vi "downloadSaved.vi"(8 "error in":errorcluster) -> (0 "error out":errorcluster, 3 "OK?":bool)   [LabVIEW 2024]
uses:
  session.vi
  user_name.vi
  <vilib>/httpClient/LabVIEWHTTPClient.lvlib
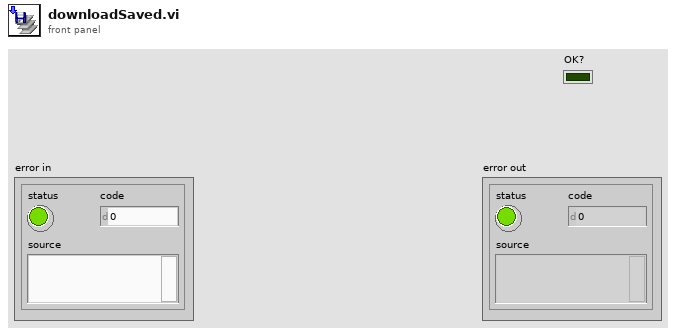
[diagram p1: front panel]
types:
  T1 = typedef "LabVIEWHTTPClient.lvlib/ClientHandle.ctl" = refnum<k1>
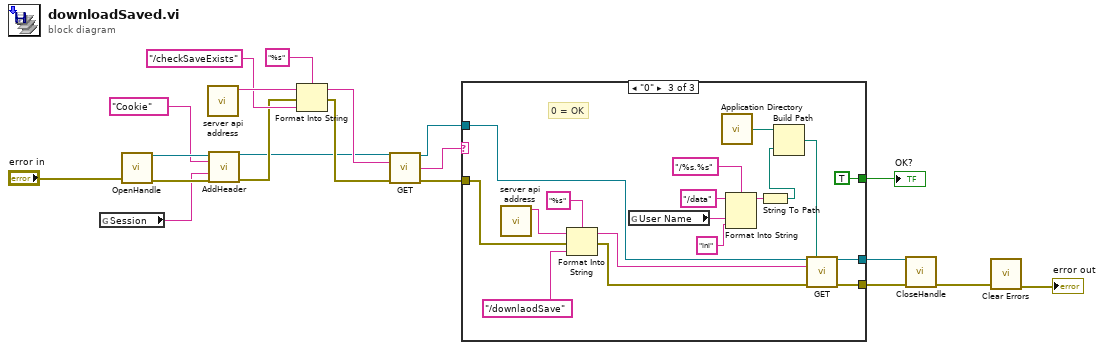
[diagram p0: block diagram]
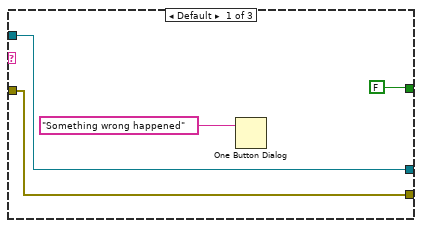
[diagram p2: hidden frame]
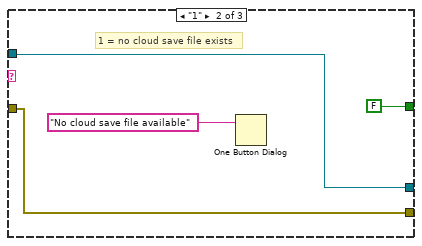
[diagram p3: hidden frame]
diagram:
  n1 = global read "session.vi" "Session"() -> (w6:string)
  n2 = call <vilib>:"OpenHandle.vi"("error in (no error)"="error in") -> ("client handle out"=w10:T1, "error out"=w11:errorcluster)  [unwired: 13 in]
  n3 = call "server api address.vi"() -> ("Server API URL"=w17:string)  [unwired: 11 in]
  n4 = call <vilib>:"AddHeader.vi"("client handle"=w10, "header"="Cookie", "value"=w6, "error in (no error)"=w11) -> ("client handle out"=w8:T1, "error out"=w9:errorcluster)  [unwired: 10 in]
  n5 = Format Into String(format string="%s", initial string=w17, error in=w9, "/checkSaveExists" ("input 1")) -> (resulting string=w15:string, error out=w18:errorcluster)
  n6 = call <vilib>:"GET.vi"("client handle"=w8, "url"=w15, "error in (no error)"=w18) -> ("client handle out"=w13:T1, "body"=w12:string, "error out"=w14:errorcluster)  [unwired: 9 in, 1 out]
  n7 = case shown="\"0\"" w12 {
    tunnel: w14 -> [w22 w27 w44]
    tunnel: w13 -> [w23 w28 w46]
    tunnel: [w23 w28 w31] -> w5
    tunnel: [w22 w27 w30] -> w4
    tunnel: [FALSE FALSE TRUE] -> w3
    frame Default {
      n8 = One Button Dialog(message="Something wrong happened") -> ()  [unwired: 1 in, 1 out]
    }
    frame "1" {
      # "1 = no cloud save file exists"
      n9 = One Button Dialog(message="No cloud save file available") -> ()  [unwired: 1 in, 1 out]
    }
    frame "0" {
      # "0 = OK"
      n10 = call "server api address.vi"() -> ("Server API URL"=w41:string)  [unwired: 11 in]
      n11 = Format Into String(format string="%s", initial string=w41, error in=w44, "/downlaodSave" ("input 1")) -> (resulting string=w42:string, error out=w43:errorcluster)
      n12 = global read "user_name.vi" "User Name"() -> (w34:string)
      n13 = call <vilib>:"Application Directory.vi"() -> ("Application Directory"=w33:path)
      n14 = Format Into String(format string="/%s.%s", initial string="/data", w34, "ini" ("input 2")) -> (resulting string=w38:string)  [unwired: 1 in, 1 out]
      n15 = String To Path(string=w38) -> (path=w37:path)
      n16 = Build Path(base path=w33, name or relative path=w37) -> (appended path=w39:path)
      n17 = call <vilib>:"GET.vi"("client handle"=w46, "output file"=w39, "url"=w42, "error in (no error)"=w43) -> ("client handle out"=w31:T1, "error out"=w30:errorcluster)  [unwired: 8 in, 2 out]
    }
  }
  "OK?" <- w3
  n18 = call <vilib>:"CloseHandle.vi"("client handle"=w5, "error in (no error)"=w4) -> ("error out"=w2:errorcluster)  [unwired: 13 in]
  n19 = call <vilib>:"Clear Errors.vi"("error in (no error)"=w2) -> ("error out"=→"error out":errorcluster)  [unwired: 5 in, 1 out]
